vi "FindTimeAtKeyTemperatures.vi"(10 "time stamps":timestamp[](array[timestamp])=array[23355 elements], 11 "ReferenceTemperature":dbl[](array[numeric])=array[23355 elements]) -> ()   [LabVIEW 2024]
uses:
  controls/KeyTempDefinition.ctl
  controls/TempFeature.ctl
  <vilib>/Utility/miscctls.llb/LVCursorListTypeDef.ctl
  <vilib>/measure/mamon.llb/Trigger Detection for 1 Channel.vi
  <vilib>/measure/NI_MAPro.lvlib
panel:
  out "Array":dbl[](array[numeric])
  in  "Key Temperatures":T1[](array[typedef])
  out "Temp Graph":waveform(dbl)(graph)={"t0"=timestamp(3821517122.4112234 s since 1904-01-01), "dt"=1.0, "Y"=array[23355 elements]}
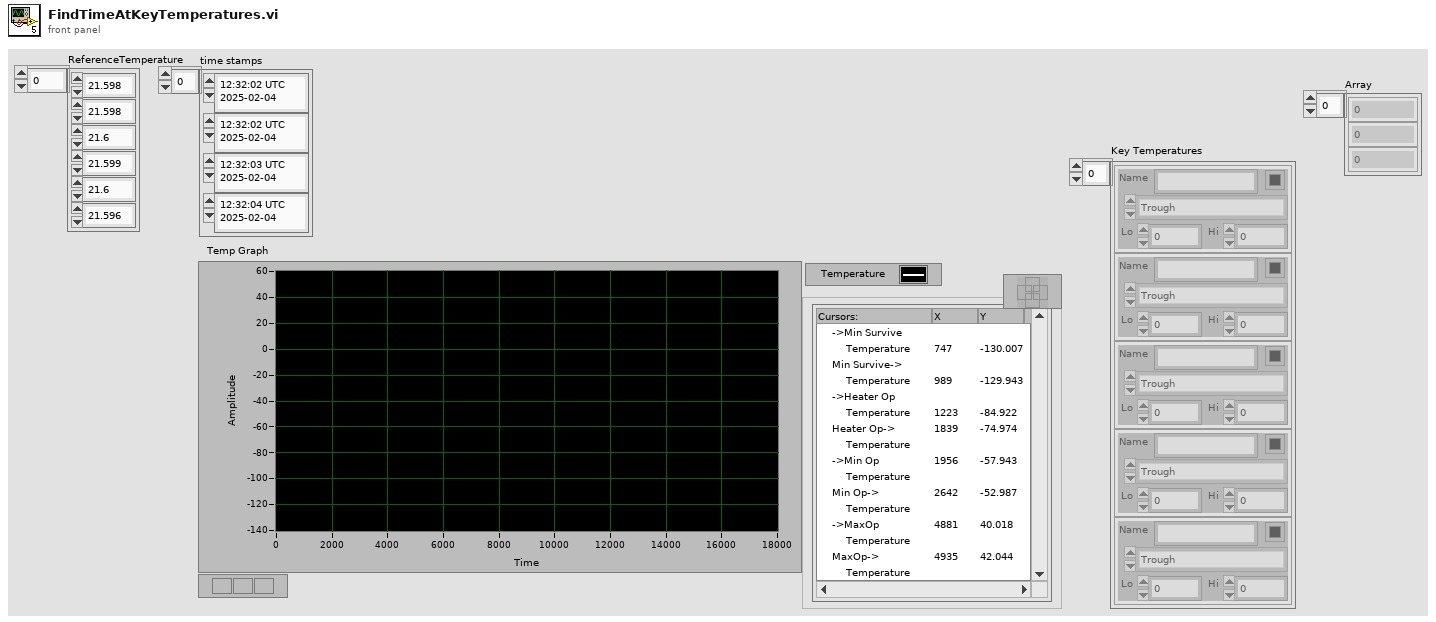
[diagram p1: front panel]
types:
  T1 = typedef "KeyTempDefinition.ctl" = cluster{"Name":string, "Feature":T2, "Lo":dbl, "Hi":dbl, "Cursor":u32}
  T2 = typedef "TempFeature.ctl" = enum16{"Trough", "Shelf Up", "Shelf Down", "Peak"}
  T3 = typedef "LVCursorListTypeDef.ctl" = cluster{"Name":string, "Color":u32, "Style":u8, "Point Style":u8, "Name Visible":bool, "Allow Drag":bool, "Cursor Mode":u32, "Plot":i32, "Index":i32, "Position":cluster{"X":dbl, "Y":dbl}, "X Scale":u32, "Y Scale":u32, "Watch Plots":i32[], "Watch All Plots":bool, "Plot Area":i32, "Label Offset":cluster{"X":dbl, "Y":dbl}}[]
  T4 = cluster{"Name":string, "Color":u32, "Style":u8, "Point Style":u8, "Name Visible":bool, "Allow Drag":bool, "Cursor Mode":u32, "Plot":i32, "Index":i32, "Position":cluster{"X":dbl, "Y":dbl}, "X Scale":u32, "Y Scale":u32, "Watch Plots":i32[], "Watch All Plots":bool, "Plot Area":i32, "Label Offset":cluster{"X":dbl, "Y":dbl}}
  T5 = cluster{"Name":string, "Color":u32, "Style":u8, "Point Style":u8, "Name Visible":bool, "Allow Drag":bool, "Cursor Mode":u32, "Plot":i32, "Index":i32, "Position":cluster{"X":dbl, "Y":dbl}, "X Scale":u32, "Y Scale":u32, "Watch Plots":i32[], "Watch All Plots":bool, "Plot Area":i32, "Label Offset":cluster{"X":dbl, "Y":dbl}}[]
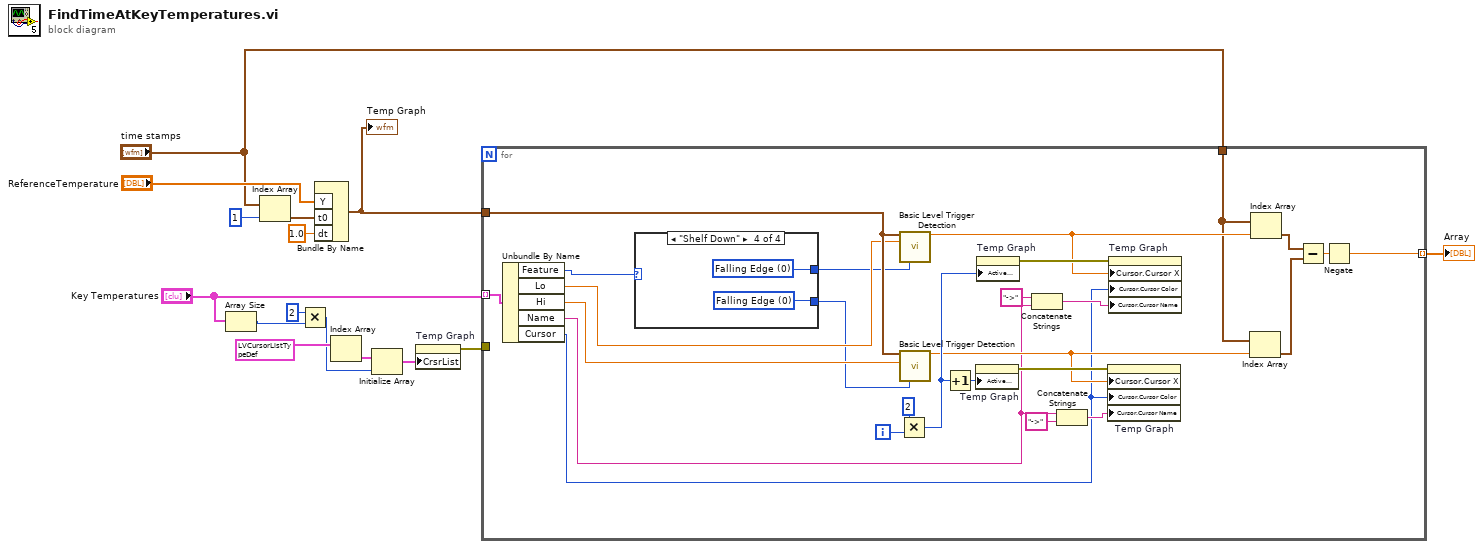
[diagram p0: block diagram]
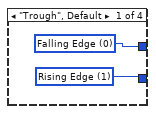
[diagram p2: hidden frame]
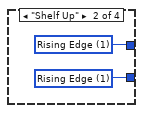
[diagram p3: hidden frame]
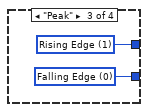
[diagram p4: hidden frame]
diagram:
  n1 = Array Size(array="Key Temperatures") -> (size(s)=w6:i32)
  n2 = Index Array(array="time stamps", index=1) -> (element=w12:timestamp)
  n3 = Multiply(x=2, y=w6) -> (x*y=w2:i32)
  n4 = Bundle By Name("Y"="ReferenceTemperature", "t0"=w12, "dt"=1.0) -> (w11:waveform(dbl))  [unwired: 1 in]
  "Temp Graph" <- w11
  n5 = Index Array(array=T3 [{"Name"="->MinSurv", "Color"=9567230, "Style"=2, "Point Style"=13, "Name Visible"=FALSE, "Allow Drag"=TRUE, "Cursor Mode"=1, "Plot"=-1, "Index"=5075, "Position"={"X"=5075.0, "Y"=-130.0}, "X Scale"=0, "Y Scale"=0, "Watch Plots"=[], "Watch All Plots"=FALSE, "Plot Area"=0, "Label Offset"={"X"=2.8443113772455035, "Y"=13.629343629343623}}, {"Name"="<-MinSurv", "Color"=9567230, "Style"=2, "Point Style"=13, "Name Visible"=FALSE, "Allow Drag"=TRUE, "Cursor Mode"=1, "Plot"=-1, "Index"=6387, "Position"={"X"=6387.0, "Y"=-129.987}, "X Scale"=0, "Y Scale"=0, "Watch Plots"=[], "Watch All Plots"=FALSE, "Plot Area"=0, "Label Offset"={"X"=-15.742514970059347, "Y"=13.616343629343618}}, {"Name"="->HtrLo", "Color"=16711680, "Style"=2, "Point Style"=13, "Name Visible"=FALSE, "Allow Drag"=TRUE, "Cursor Mode"=1, "Plot"=-1, "Index"=7571, "Position"={"X"=7571.0, "Y"=-84.98}, "X Scale"=0, "Y Scale"=0, "Watch Plots"=[], "Watch All Plots"=FALSE, "Plot Area"=0, "Label Offset"={"X"=-2.1377245508983833, "Y"=13.783088803088816}}, {"Name"="->HtrHi", "Color"=16711680, "Style"=2, "Point Style"=13, "Name Visible"=FALSE, "Allow Drag"=TRUE, "Cursor Mode"=1, "Plot"=-1, "Index"=10398, "Position"={"X"=10398.0, "Y"=-74.976}, "X Scale"=0, "Y Scale"=0, "Watch Plots"=[], "Watch All Plots"=FALSE, "Plot Area"=0, "Label Offset"={"X"=-2.7904191616762546, "Y"=14.203799227799237}}, {"Name"="Cursor 4", "Color"=16776960, "Style"=2, "Point Style"=13, "Name Visible"=FALSE, "Allow Drag"=TRUE, "Cursor Mode"=1, "Plot"=-1, "Index"=11161, "Position"={"X"=11161.0, "Y"=-55.0}, "X Scale"=0, "Y Scale"=0, "Watch Plots"=[], "Watch All Plots"=FALSE, "Plot Area"=0, "Label Offset"={"X"=0.6766467065863253, "Y"=13.68725868725869}}, {"Name"="Cursor 5", "Color"=16776960, "Style"=2, "Point Style"=13, "Name Visible"=FALSE, "Allow Drag"=TRUE, "Cursor Mode"=1, "Plot"=-1, "Index"=14279, "Position"={"X"=14279.0, "Y"=-51.993}, "X Scale"=0, "Y Scale"=0, "Watch Plots"=[], "Watch All Plots"=FALSE, "Plot Area"=0, "Label Offset"={"X"=-3.5508982035917143, "Y"=14.155162162162178}}] ("Cursor List")) -> (element=w7:T4)  [unwired: 1 in]
  n6 = Initialize Array(w7, w2) -> (w5:T5)
  n7 = property on="Temp Graph" class="WFGraph (strict)"("CrsrList"=w5) -> (error out=w4:errorcluster)  [unwired: 2 in, 1 out]
  n8 = for {
    tunnel: "Key Temperatures" -> [w41] mode=indexing
    tunnel: w11 -> [w40]
    tunnel: "time stamps" -> [w29]
    tunnel: [w20] -> w9 mode=indexing
    tunnel: w4 -> [_]
    i -> [w37]
    n9 = Unbundle By Name(w41) -> ("Feature"=w18:T2, "Lo"=w39:dbl, "Hi"=w38:dbl, "Name"=w25:string, "Cursor"=w19:u32)
    n10 = case shown="\"Shelf Down\"" w18 {
      tunnel: [w43 w45 w46 w49] -> w17
      tunnel: [w42 w44 w47 w48] -> w16
      frame "Trough", Default {
        w42 = u16 1 items=["Falling Edge", "Rising Edge"] ("trigger slope 2")
        w43 = u16 0 items=["Falling Edge", "Rising Edge"] ("trigger slope")
      }
      frame "Shelf Up" {
        w44 = u16 1 items=["Falling Edge", "Rising Edge"] ("trigger slope 2")
        w45 = u16 1 items=["Falling Edge", "Rising Edge"] ("trigger slope")
      }
      frame "Peak" {
        w46 = u16 1 items=["Falling Edge", "Rising Edge"] ("trigger slope")
        w47 = u16 0 items=["Falling Edge", "Rising Edge"] ("trigger slope")
      }
      frame "Shelf Down" {
        w48 = u16 0 items=["Falling Edge", "Rising Edge"] ("trigger slope")
        w49 = u16 0 items=["Falling Edge", "Rising Edge"] ("trigger slope")
      }
    }
    n11 = Multiply(x=2, y=w37) -> (x*y=w32:i32)
    n12 = call-poly <vilib>:"Basic Level Trigger Detection.vi"("signal in"=w40, "level"=w39, "trigger slope"=w17) -> ("trigger location"=w31:dbl)  [unwired: 10 in, 2 out]
    n13 = call-poly <vilib>:"Basic Level Trigger Detection.vi"("signal in"=w40, "level"=w38, "trigger slope"=w16) -> ("trigger location"=w30:dbl)  [unwired: 10 in, 2 out]
    n14 = Increment(x=w32) -> (x+1=w33:i32)
    n15 = property on="Temp Graph" class="WFGraph (strict)"("Active Cursor"=w33) -> (error out=w34:errorcluster)  [unwired: 2 in, 1 out]
    n16 = property on="Temp Graph" class="WFGraph (strict)"("Active Cursor"=w32) -> (error out=w35:errorcluster)  [unwired: 2 in, 1 out]
    n17 = Concatenate Strings("->" ("string"), w25) -> (w22:string)
    n18 = Concatenate Strings(w25, "->" ("string")) -> (w24:string)
    n19 = property on="Temp Graph" class="WFGraph (strict)"(error in=w34, "Cursor.Cursor X"=w30, "Cursor.Cursor Color"=w19, "Cursor.Cursor Name"=w24) -> ()  [unwired: 1 in, 2 out]
    n20 = property on="Temp Graph" class="WFGraph (strict)"(error in=w35, "Cursor.Cursor X"=w31, "Cursor.Cursor Color"=w19, "Cursor.Cursor Name"=w22) -> ()  [unwired: 1 in, 2 out]
    n21 = Index Array(array=w29, index=w30) -> (element=w27:timestamp)
    n22 = Index Array(array=w29, index=w31) -> (element=w28:timestamp)
    n23 = Subtract(x=w28, y=w27) -> (x-y=w26:dbl)
    n24 = Negate(x=w26) -> (-x=w20:dbl)
  }
  "Array" <- w9
